vi "Add NI-XNET CAN Hardware.vi"(7 "Overwrite Existing?":bool=TRUE, 8 "error in (no error)":errorcluster, 9 "CAN Settings":T1={"Name"="", "Database Name"="", "PortNumber"=0, "ClusterName"="", "BaudRate"=500000, "InlineIncoming"=FALSE, "IncomingRate"=100, "InlineOutgoing"=FALSE, "OutgoingRate"=100, "Termination"=0, "Echo"=FALSE, "InputStreamQueueSize"=120000, "CANBusOff"=FALSE, "CANBusOffRate"=1, "TransceiverType"=0, "TransmitOrderType"=0, "Cyclic Frames"=[], "Outgoing Frames"=[], "Incoming Frames"=[], "Log Files"=[]} {"Log Files"."Operation" items=["ContinueLoggingInNewFile", "StopLogging"]; "Log Files"."LimitType" items=["Footprint", "Time"]; "Log Files"."TriggerType" items=["StartLoggingOnNonZero", "StartLoggingOnZero", "EnableLoggingWhenTriggerIsZero", "EnableLoggingWhenTriggerIsNonZero"]; "Log Files"."Filter" items=["LogEntireBusTraffic", "ExcludeFrameIDs", "IncludeFrameIDs"]; "Log Files"."DataLoggingFileType" items=["TDMS", "NCL"]; "TransmitOrderType" items=["AsSubmitted", "ByIdentifier"]; "TransceiverType" items=["HS", "LS", "SW"]; "Termination" items=["Off", "On"]; "Outgoing Frames"."Phase" items=["Unchanged", "Reset"]; "Outgoing Frames"."TriggerType" items=["ChannelValueChange", "TriggerChannelNotZero", "ChannelValueChangeOrTriggerChannelNotZero"]}, 10 "Base Node Path":string, 11 "SysDef Ref":T7) -> (0 "error out":errorcluster, 2 "New Node Path":string, 3 "SysDef Ref Out":T7)   [LabVIEW 2019, in "Simple SysDef API.lvlib"]
uses:
  <userlib>/SimpleSysDef/Simple SysDef API.lvlib
  <userlib>/SimpleSysDef/_SubVIs/System Definition Reference.ctl
  NationalInstruments.VeriStand.SystemDefinitionAPI
  <userlib>/SimpleSysDef/_SubVIs/Add NI-XNET CAN Hardware_Port Settings.ctl
  <userlib>/SimpleSysDef/_SubVIs/Add NI-XNET CAN Hardware_Periodic Frame Settings.ctl
  <userlib>/SimpleSysDef/_SubVIs/Add NI-XNET CAN Hardware_Frame Settings.ctl
  <userlib>/SimpleSysDef/_SubVIs/Add NI-XNET CAN Hardware_Signal Settings.ctl
  <userlib>/SimpleSysDef/_SubVIs/Add NI-XNET CAN Hardware_Sporadic Frame Settings.ctl
  <userlib>/SimpleSysDef/_SubVIs/Add NI-XNET CAN Hardware_Add Log File_Settings.ctl
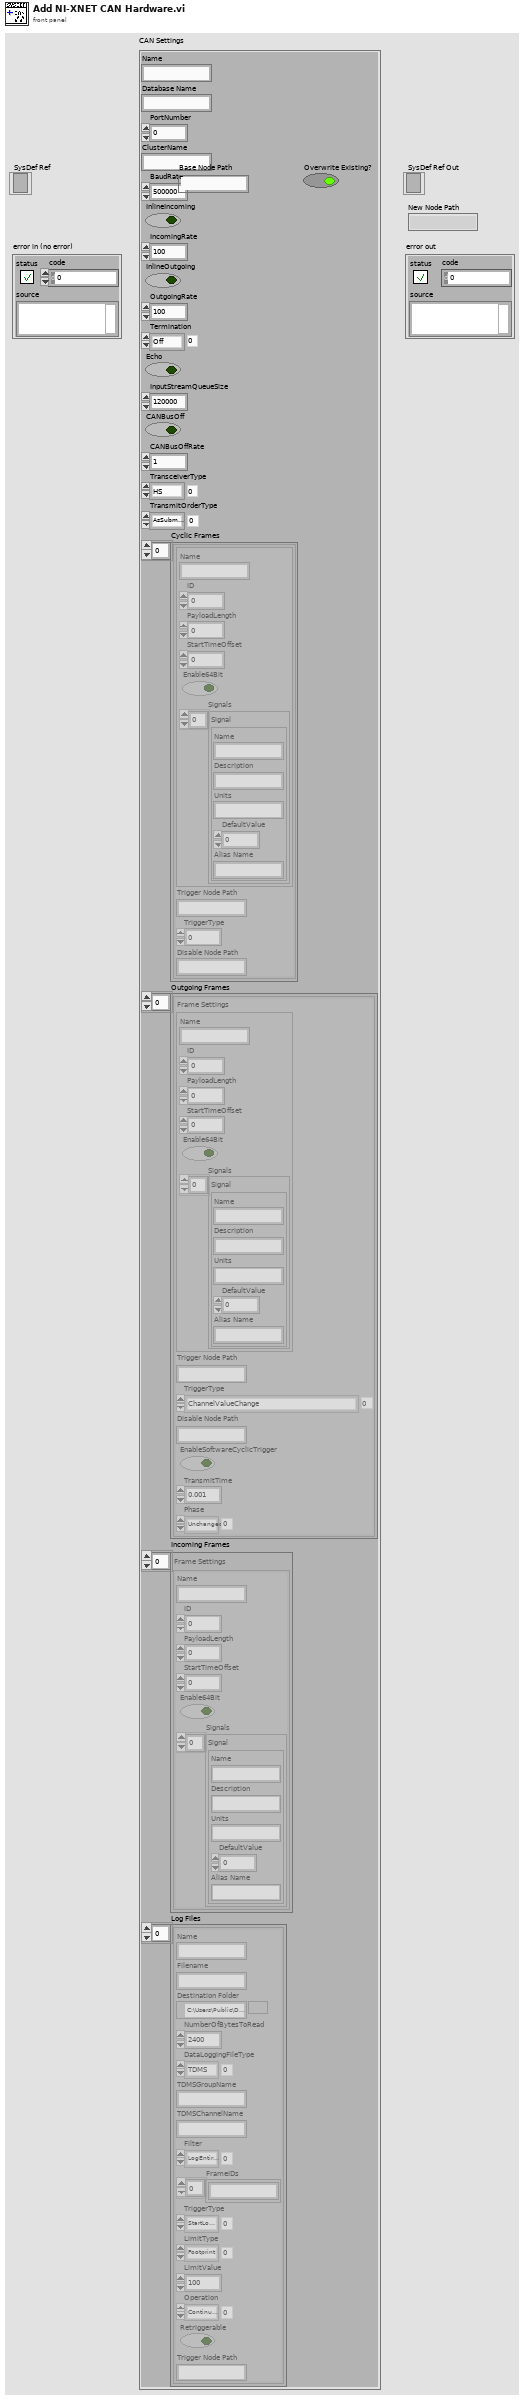
[diagram p1: front panel]
types:
  T1 = typedef "Simple SysDef API.lvlib/Add NI-XNET CAN Hardware_Port Settings.ctl" = cluster{"Name":string, "Database Name":string, "PortNumber":u16, "ClusterName":string, "BaudRate":u32, "InlineIncoming":bool, "IncomingRate":u32, "InlineOutgoing":bool, "OutgoingRate":u32, "Termination":i32, "Echo":bool, "InputStreamQueueSize":u32, "CANBusOff":bool, "CANBusOffRate":u32, "TransceiverType":i32, "TransmitOrderType":i32, "Cyclic Frames":T2[], "Outgoing Frames":T5[], "Incoming Frames":T3[], "Log Files":T6[]}
  T2 = typedef "Simple SysDef API.lvlib/Add NI-XNET CAN Hardware_Periodic Frame Settings.ctl" = cluster{"Frame Settings":T3, "Trigger Node Path":string, "TriggerType":i32, "Disable Node Path":string}
  T3 = typedef "Simple SysDef API.lvlib/Add NI-XNET CAN Hardware_Frame Settings.ctl" = cluster{"Name":string, "ID":u32, "PayloadLength":u32, "StartTimeOffset":dbl, "Enable64Bit":bool, "Signals":T4[]}
  T4 = typedef "Simple SysDef API.lvlib/Add NI-XNET CAN Hardware_Signal Settings.ctl" = cluster{"Name":string, "Description":string, "Units":string, "DefaultValue":dbl, "Alias Name":string}
  T5 = typedef "Simple SysDef API.lvlib/Add NI-XNET CAN Hardware_Sporadic Frame Settings.ctl" = cluster{"Frame Settings":T3, "Trigger Node Path":string, "TriggerType":i32, "Disable Node Path":string, "EnableSoftwareCyclicTrigger":bool, "TransmitTime":dbl, "Phase":i32}
  T6 = typedef "Simple SysDef API.lvlib/Add NI-XNET CAN Hardware_Add Log File_Settings.ctl" = cluster{"Name":string, "Filename":string, "Destination Folder":path, "NumberOfBytesToRead":u32, "DataLoggingFileType":i32, "TDMSGroupName":string, "TDMSChannelName":string, "Filter":i32, "FrameIDs":string[], "TriggerType":i32, "LimitType":i32, "LimitValue":u32, "Operation":i32, "Retriggerable":bool, "Trigger Node Path":string}
  T7 = typedef "Simple SysDef API.lvlib/System Definition Reference.ctl" = refnum<k24>
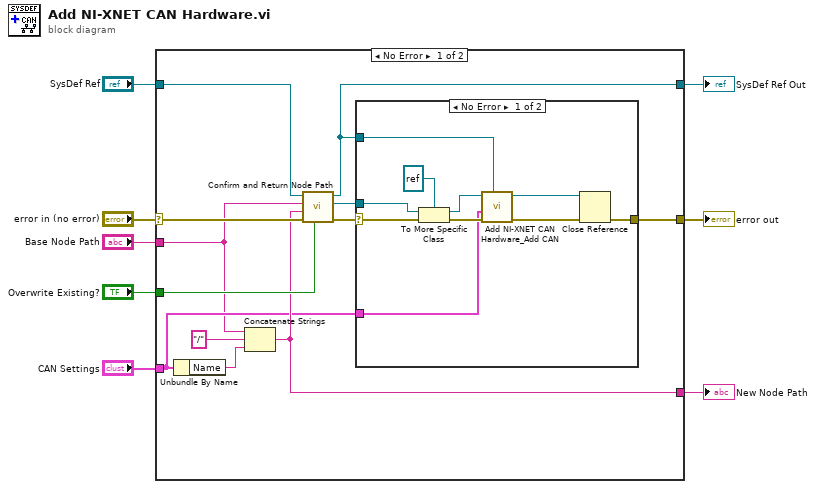
[diagram p0: block diagram]
diagram:
  n1 = case shown="No Error" "error in (no error)" {
    selector: "error in (no error)" -> [w20 w33]
    tunnel: [w16 w33] -> w7
    tunnel: "SysDef Ref" -> [w19 w32]
    tunnel: [w11 w32] -> w5
    tunnel: "Base Node Path" -> [w9 _]
    tunnel: "Overwrite Existing?" -> [w13 _]
    tunnel: "CAN Settings" -> [w10 _]
    tunnel: [w12 _] -> w1
    frame No Error {
      n2 = Unbundle By Name(w10) -> ("Name"=w17:string)
      n3 = Concatenate Strings(w9, "/" ("string"), w17) -> (w12:string)
      n4 = call <userlib>:"Confirm and Return Node Path.vi"("Overwrite Existing?"=w13, "error in (no error)"=w20, "New Node Path"=w12, "Base Node Path"=w9, "SysDef Ref"=w19) -> ("error out"=w14:errorcluster, "Node Ref"=w15:refnum<k24>, "SysDef Ref Out"=w11:T7)  [unwired: 4 in]
      n5 = case shown="No Error" w14 {
        selector: w14 -> [w29 w31]
        tunnel: [w28 w31] -> w16
        tunnel: w15 -> [w30 _]
        tunnel: w11 -> [w26 _]
        tunnel: w10 -> [w22 _]
        frame No Error {
          n6 = To More Specific Class(target class=refnum<k24> refnum ("Node Ref"), reference=w30, error in=w29) -> (specific class reference=w21:refnum<k24>, error out=w24:errorcluster)
          n7 = call <userlib>:"Add NI-XNET CAN Hardware_Add CAN.vi"("SysDef Ref"=w26, "error in (no error)"=w24, "CAN Settings"=w22, "CAN Ref"=w21) -> ("error out"=w23:errorcluster, "CAN Ref Out"=w25:refnum<k24>)  [unwired: 6 in]
          n8 = Close Reference(reference=w25, error in (no error)=w23) -> (error out=w28:errorcluster)
        }
        frame Error {
        }
      }
    }
    frame Error {
    }
  }
  "SysDef Ref Out" <- w5
  "error out" <- w7
  "New Node Path" <- w1
